vi "mupSetVarValue.vi"(8 "error in (no error)":errorcluster, 10 "varValue":dbl, 11 "varPtr in":u64) -> (0 "error out":errorcluster, 3 "varPtr out":u64)   [LabVIEW 2015, in "muParser.lvlib"]
uses:
  muParser.lvlib
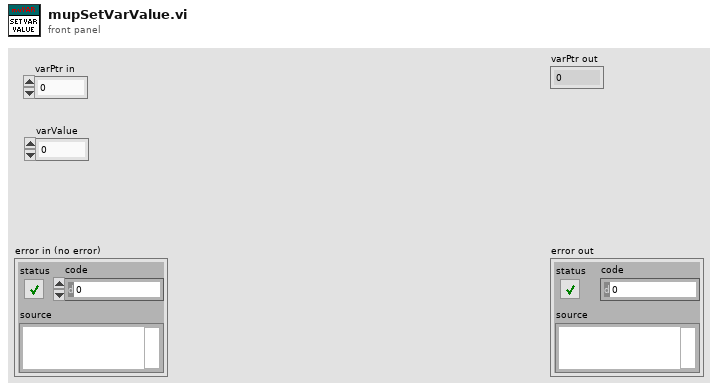
[diagram p1: front panel]
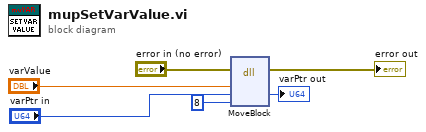
[diagram p0: block diagram]
diagram:
  n1 = dll-call lib="LabVIEW" fn="MoveBlock"(error in="error in (no error)", "ps"="varValue", "pd"="varPtr in", "size"=8) -> (error out=→"error out":errorcluster, "pd"=→"varPtr out":u64)  [unwired: 5 in, 1 out]
